vi "ACC_LabVIEW_Call_Example.vi"() -> ()   [LabVIEW 2014, in "ACC_LabVIEW.lvlib"]
doc: "Example for using the \"call\" method."
uses:
  ACC_LabVIEW.lvlib
panel:
  in  "VirtAcc":i32
  out "error out":errorcluster
  in  "Propname":string="INIT"
  in  "Nomenklatur":string="K4XCS012"
  # "Please mention:\n\nA read-action wil work every time on every device. But to perform a \"write\" or \"call\" , you need \nto be registered inside the \"right.xml\" file of the nameserver.\nTo get this managed, ask Solveigh Matthies from the BEL - department."
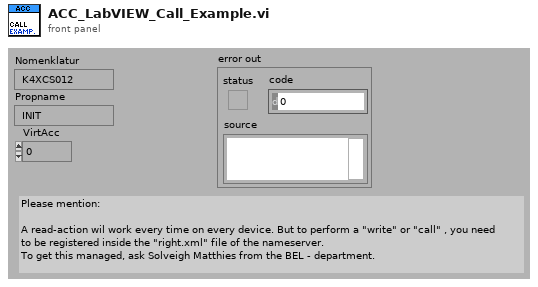
[diagram p1: front panel]
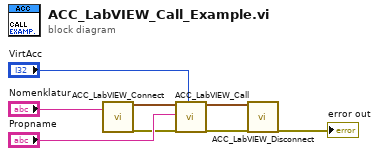
[diagram p0: block diagram]
diagram:
  n1 = call "ACC_LabVIEW_Connect.vi"("Nomenklatur"="Nomenklatur") -> ("DeviceReferenceOut"=w2:cluster{"ID":u32}, "error out"=w6:errorcluster)  [unwired: 17 in]
  n2 = call "ACC_LabVIEW_Call.vi"("DeviceReferenceIn"=w2, "Propname"="Propname", "error in (no error)"=w6, "VirtAcc"="VirtAcc") -> ("DeviceReferenceOut"=w1:cluster{"ID":u32}, "error out"=w5:errorcluster)  [unwired: 14 in]
  n3 = call "ACC_LabVIEW_Disconnect.vi"("DeviceReferenceIn"=w1, "error in (no error)"=w5) -> ("error out"=→"error out":errorcluster)  [unwired: 17 in]
